vi "PH_Beckhoff_PP_Control.handle PP Mercury.vi"(0 "i ref in":refnum<vi>, 1 "changed DE Values":i32[](array[numeric]), 2 "changed AE Values":i32[](array[numeric]), 3 "Current Digital Inputs":T3, 4 "Current Analog Inputs":T1, 5 "error in":errorcluster) -> (14 "i ref out":refnum<vi>, 19 "error out":errorcluster)   [LabVIEW 2014, in "PH_Beckhoff_PP_Control.lvlib"]
doc: "This VI handles all information related to the PP mercury measurement. If it changed, it publishes the current status, the time since running, and sets the related GUI element."
uses:
  PH_Beckhoff_PP_Control.lvlib
  PH_Beckhoff/PH_Beckhoff.Digital Inputs.ctl
  PH_Beckhoff/PH_Beckhoff.Analog Inputs.ctl
  PH_Beckhoff/PH_Beckhoff.Scaling Type.ctl
  PH_StatusHandler/PH_StatusHandler.Status.ctl
  PH_StatusHandler/PH_StatusHandler.lvlib
  lib.lib/DimLVEvent/LVDimInterface/LVDimInterface.lvlib
  PH_Common/PH_Common.lvlib
  PH_Beckhoff/PH_Beckhoff.lvlib
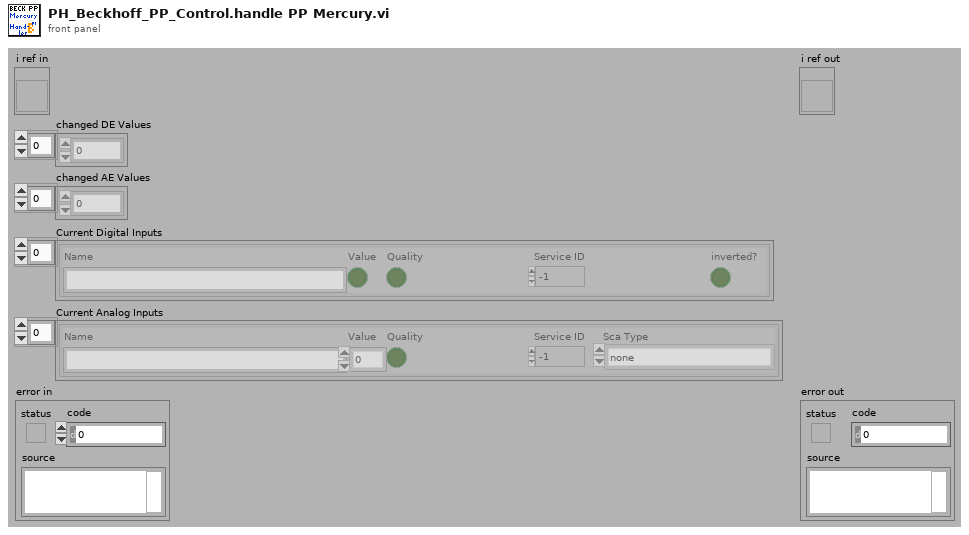
[diagram p1: front panel]
types:
  T1 = typedef "PH_Beckhoff.lvlib/PH_Beckhoff.Analog Inputs.ctl" = cluster{"Name":string, "Value":u32, "Quality":bool, "Service ID":i32, "Sca Type":T2}[]
  T2 = typedef "PH_Beckhoff.lvlib/PH_Beckhoff.Scaling Type.ctl" = enum16{"none", "0 ... 15 Bit -> 0 ... 5", "0 ... 15 Bit -> 0 ... 10", "0 ... 15 Bit -> 0 ... 25", "0 ... 15 Bit -> 4 ... 20", "0 ... 15 Bit -> 0 ... 1", "0 ... 15 Bit -> 0 ... 20000", "0 ... 15 Bit -> 0 ... 24000"}
  T3 = typedef "PH_Beckhoff.lvlib/PH_Beckhoff.Digital Inputs.ctl" = cluster{"Name":string, "Value":bool, "Quality":bool, "Service ID":i32, "inverted?":bool}[]
  T4 = typedef "PH_Beckhoff_PP_Control.lvlib/PH_Beckhoff_PP_Control.i attribute.ctl" = cluster{"PP Conductivity Control":cluster{"PSDB":cluster{"Status Service ID":i32, "Instance ID":i32, "Data Status":T5, "Ref Status":refnum<vi>, "Error Code":i32}, "Status":cluster{"GUI Ref":refnum<vi>, "Status Service ID":i32, "Status":T6}, "DIs":cluster{"Device on":cluster{"GUI Ref":refnum<vi>, "# in Data":i32}, "Conductivity ok":cluster{"GUI Ref":refnum<vi>, "# in Data":i32}, "Temperature ok":cluster{"GUI Ref":refnum<vi>, "# in Data":i32}, "Alarm":cluster{"GUI Ref":refnum<vi>, "# in Data":i32}}, "PSDB Thread":cluster{"Ref":refnum<vi>, "Q-Ref":refnum<queue>}}, "PP Mercury Control":cluster{"PSDB":cluster{"Status Service ID":i32, "Instance ID":i32, "Data Status":T5, "Ref Status":refnum<vi>, "Error Code":i32}, "Status":cluster{"GUI Ref":refnum<vi>, "Status Service ID":i32, "Status":T6}, "on since:":cluster{"GUI Ref":refnum<vi>, "Service ID":i32, "Time":string}, "DIs":cluster{"Device on":cluster{"GUI Ref":refnum<vi>, "# in Data":i32}, "Alarm":cluster{"GUI Ref":refnum<vi>, "# in Data":i32}}, "AIs":cluster{"Concentration":cluster{"GUI Ref":refnum<vi>, "# in Data":i32}}, "PSDB Thread":cluster{"Ref":refnum<vi>, "Q-Ref":refnum<queue>}}, "PSDB":cluster{"Shot #":i32, "Subsystem":T7}, "PSDB Credentials":T8}
  T5 = typedef "PH_PSDBWriter.lvlib/PH_PSDBWriter.Data Status.ctl" = i16
  T6 = typedef "PH_StatusHandler.lvlib/PH_StatusHandler.Status.ctl" = i16
  T7 = typedef "PH_PSDBWriter.lvlib/PH_PSDBWriter.PHELIX-Subsystems.ctl" = i32
  T8 = typedef "PH_Common.lvlib/PH_Connection.PSDB Credentials.ctl" = cluster{"PW":string, "ID":string, "DS":string}
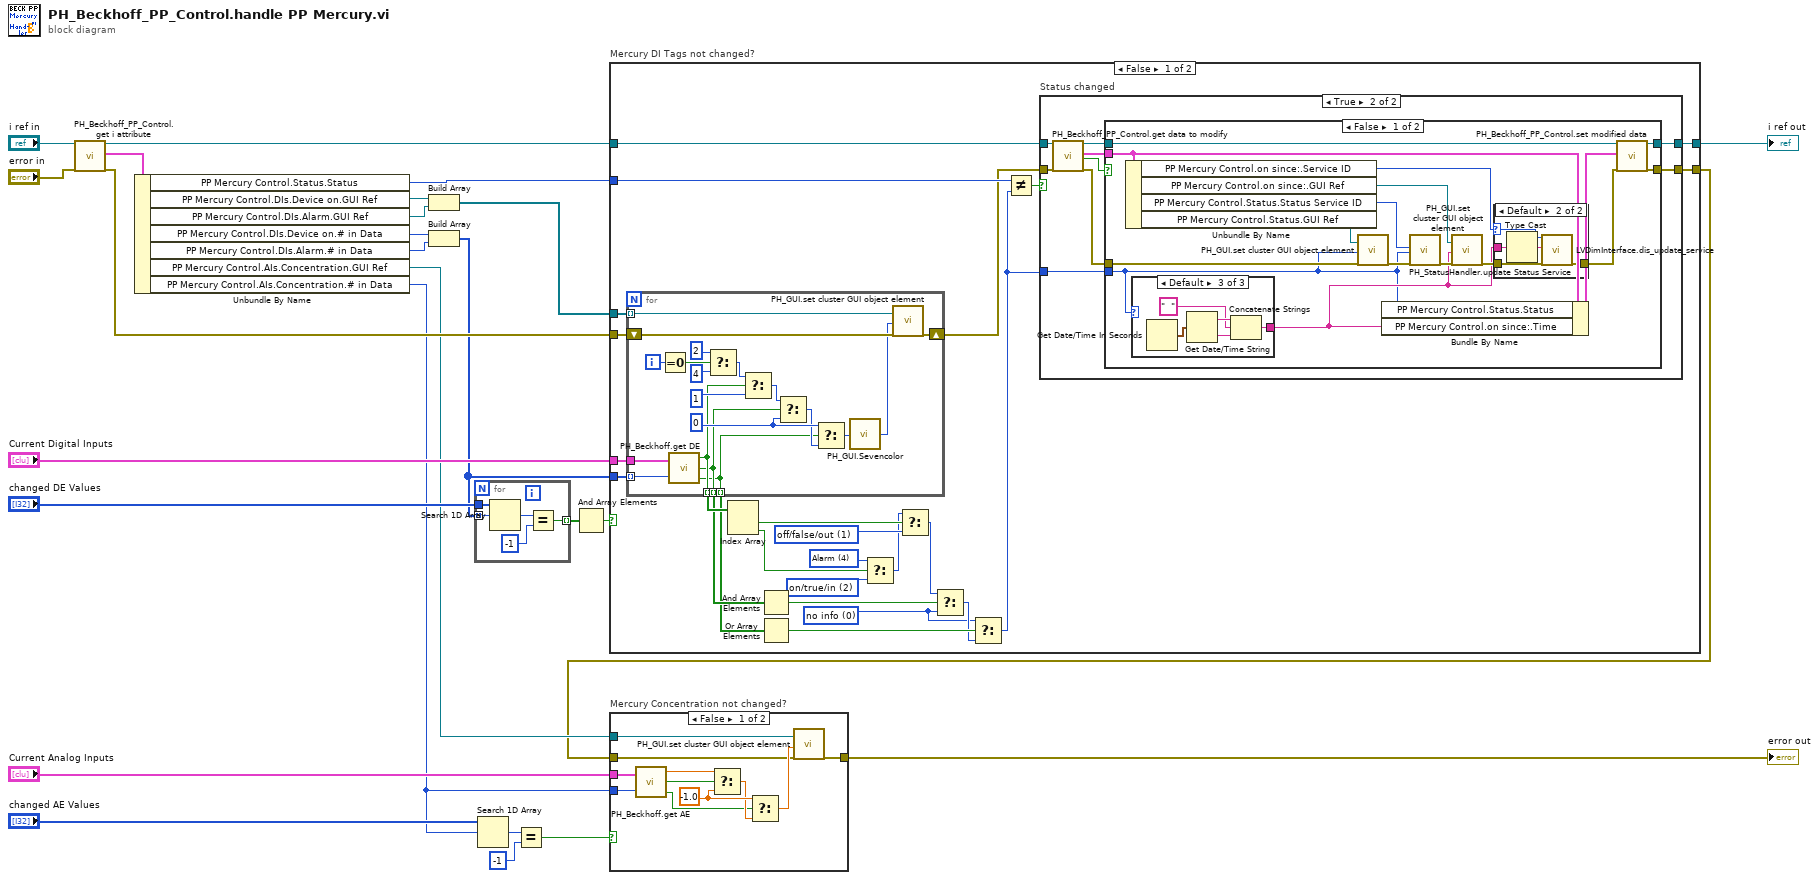
[diagram p0: block diagram]
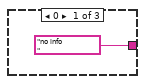
[diagram p5: hidden frame]
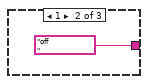
[diagram p6: hidden frame]
diagram:
  n1 = call "PH_Beckhoff_PP_Control.get i attribute.vi"("i ref in"="i ref in", "error in (no error)"="error in") -> ("i ref out"=w24:refnum<vi>, "i attribute"=w22:T4, "error out"=w13:errorcluster)  [unwired: 15 in]
  n2 = Unbundle By Name(w22) -> ("PP Mercury Control.Status.Status"=w21:T6, "PP Mercury Control.DIs.Device on.GUI Ref"=w18:refnum<vi>, "PP Mercury Control.DIs.Alarm.GUI Ref"=w17:refnum<vi>, "PP Mercury Control.DIs.Device on.# in Data"=w16:i32, "PP Mercury Control.DIs.Alarm.# in Data"=w15:i32, "PP Mercury Control.AIs.Concentration.GUI Ref"=w7:refnum<vi>, "PP Mercury Control.AIs.Concentration.# in Data"=w6:i32)
  n3 = Build Array(w18, w17) -> (w14:refnum<vi>[])
  n4 = Build Array(w16, w15) -> (w11:i32[])
  n5 = for {
    tunnel: "changed DE Values" -> [w31]
    tunnel: w11 -> [w30] mode=indexing
    tunnel: [w29] -> w10 mode=indexing
    n6 = Search 1D Array(1D array=w31, element=w30) -> (index of element=w28:i32)  [unwired: 1 in]
    n7 = Equal?(x=w28, y=-1) -> (x = y?=w29:bool)
  }
  n8 = Search 1D Array(1D array="changed AE Values", element=w6) -> (index of element=w2:i32)  [unwired: 1 in]
  n9 = Equal?(x=w2, y=-1) -> (x = y?=w3:bool)
  n10 = And Array Elements(Boolean array=w10) -> (logical AND=w9:bool)
  n11 = case "Mercury DI Tags not changed?" shown="False" w9 {
    tunnel: w24 -> [w43 w119]
    tunnel: w21 -> [w42 _]
    tunnel: [w41 w119] -> w20
    tunnel: [w40 w118] -> w5
    tunnel: "Current Digital Inputs" -> [w39 _]
    tunnel: w14 -> [w35 _]
    tunnel: w13 -> [w34 w118]
    tunnel: w11 -> [w32 _]
    frame False {
      w45 = T6 2 items=["no info", "off/false/out", "on/true/in", "Failure", "Alarm", "Status 1", "Status 2", "Status 3"] ("PP Mercury Control.Status")
      w46 = T6 4 items=["no info", "off/false/out", "on/true/in", "Failure", "Alarm", "Status 1", "Status 2", "Status 3"] ("PP Mercury Control.Status")
      w50 = T6 1 items=["no info", "off/false/out", "on/true/in", "Failure", "Alarm", "Status 1", "Status 2", "Status 3"] ("PP Mercury Control.Status")
      w52 = T6 0 items=["no info", "off/false/out", "on/true/in", "Failure", "Alarm", "Status 1", "Status 2", "Status 3"] ("PP Mercury Control.Status")
      n12 = for {
        shift-right: [w65] -> w33
        shift-left: w34 -> [w64]
        tunnel: w35 -> [w63] mode=indexing
        tunnel: w39 -> [w61]
        tunnel: [w60] -> w38 mode=indexing
        tunnel: [w59] -> w37 mode=indexing
        tunnel: [w58] -> w36 mode=indexing
        tunnel: w32 -> [w57] mode=indexing
        i -> [w70]
        w75 = 0 ("State")
        n13 = Equal To 0?(x=w70) -> (x = 0?=w69:bool)
        n14 = call "PH_Beckhoff.get DE.vi"("Digital Values"=w61, "index of element"=w57) -> ("Value"=w60:bool, "Quality"=w59:bool, "Tag not found"=w58:bool)
        n15 = Select(t=2 ("State"), s=w69, f=4) -> (s? t:f=w67:i32)
        n16 = Select(t=w67, s=w60, f=1 ("State")) -> (s? t:f=w71:i32)
        n17 = Select(t=w71, s=w59, f=w75) -> (s? t:f=w74:i32)
        n18 = Select(t=w75, s=w58, f=w74) -> (s? t:f=w73:i32)
        n19 = call "PH_GUI.Sevencolor.vi"("State"=w73) -> ("Color Box"=w62:u32)
        n20 = call "PH_GUI.set cluster GUI object element.vi"("Ctl Refnum"=w63, "Value"=w62, "error in"=w64) -> ("error out"=w65:errorcluster)  [unwired: 16 in]
      }
      n21 = Index Array(array=w38) -> (element #1=w51:bool, element #2=w48:bool)  [unwired: 2 in]
      n22 = And Array Elements(Boolean array=w37) -> (logical AND=w54:bool)
      n23 = Or Array Elements(Boolean array=w36) -> (logical OR=w55:bool)
      n24 = Select(t=w46, s=w48, f=w45) -> (s? t:f=w47:T6)
      n25 = Select(t=w47, s=w51, f=w50) -> (s? t:f=w49:T6)
      n26 = Select(t=w49, s=w54, f=w52) -> (s? t:f=w53:T6)
      n27 = Select(t=w52, s=w55, f=w53) -> (s? t:f=w44:T6)
      n28 = Not Equal?(x=w42, y=w44) -> (x != y?=w56:bool)
      n29 = case "Status changed" shown="True" w56 {
        tunnel: w33 -> [w76 w86]
        tunnel: [w76 w84] -> w40
        tunnel: w43 -> [w77 w83]
        tunnel: [w77 w81] -> w41
        tunnel: w44 -> [_ w78]
        frame False {
        }
        frame True {
          n30 = call "PH_Beckhoff_PP_Control.get data to modify.vi"("i ref in"=w83, "error in (no error)"=w86) -> ("i ref out"=w82:refnum<vi>, "i attribute"=w79:T4, "timed out"=w80:bool, "error out"=w85:errorcluster)  [unwired: 14 in]
          n31 = case shown="False" w80 {
            tunnel: w85 -> [w90 w116]
            tunnel: [w102 w116] -> w84
            tunnel: w82 -> [w101 w117]
            tunnel: [w100 w117] -> w81
            tunnel: w79 -> [w98 _]
            tunnel: w78 -> [w87 _]
            frame False {
              n32 = Unbundle By Name(w98) -> ("PP Mercury Control.on since:.Service ID"=w96:i32, "PP Mercury Control.on since:.GUI Ref"=w91:refnum<vi>, "PP Mercury Control.Status.Status Service ID"=w97:i32, "PP Mercury Control.Status.GUI Ref"=w88:refnum<vi>)
              n33 = case shown="Default" w87 {
                tunnel: ["no info                              " "off                                  " w112] -> w92
                frame 0 {
                }
                frame 1 {
                }
                frame Default {
                  n34 = Get Date/Time In Seconds() -> (seconds since 1Jan1904=w111:timestamp)
                  n35 = Get Date/Time String(seconds (now)=w111) -> (date string=w115:string, time string=w114:string)  [unwired: 2 in]
                  n36 = Concatenate Strings(w115, "  " ("string"), w114) -> (w112:string)
                }
              }
              n37 = call "PH_GUI.set cluster GUI object element.vi"("Ctl Refnum"=w88, "Value"=w87, "error in"=w90) -> ("error out"=w89:errorcluster)  [unwired: 16 in]
              n38 = Bundle By Name(cluster=w98, "PP Mercury Control.Status.Status"=w87, "PP Mercury Control.on since:.Time"=w92) -> (w99:T4)
              n39 = call "PH_StatusHandler.update Status Service.vi"("Service ID"=w97, "Status"=w87, "error in (no error)"=w89) -> ("error out"=w95:errorcluster)  [unwired: 16 in]
              n40 = call "PH_GUI.set cluster GUI object element.vi"("Ctl Refnum"=w91, "Value"=w92, "error in"=w95) -> ("error out"=w93:errorcluster)  [unwired: 16 in]
              n41 = case shown="Default" w96 {
                selector: w96 -> [_ w107]
                tunnel: [w103 w104] -> w94
                tunnel: w93 -> [w103 w108]
                tunnel: w92 -> [_ w105]
                frame -1 {
                }
                frame Default {
                  n42 = Type Cast(x=w105) -> (*(type *) &x=w106:string)  [unwired: 1 in]
                  n43 = call "LVDimInterface.dis_update_service.vi"("my_serviceID"=w107, "data"=w106, "error in (no error)"=w108) -> ("error out"=w104:errorcluster)  [unwired: 14 in, 2 out]
                }
              }
              n44 = call "PH_Beckhoff_PP_Control.set modified data.vi"("i ref in"=w101, "i attribute"=w99, "error in (no error)"=w94) -> ("i ref out"=w100:refnum<vi>, "error out"=w102:errorcluster)  [unwired: 15 in]
            }
            frame True {
            }
          }
        }
      }
    }
    frame True {
    }
  }
  "i ref out" <- w20
  n45 = case "Mercury Concentration not changed?" shown="False" w3 {
    tunnel: "Current Analog Inputs" -> [w130 _]
    tunnel: w7 -> [w123 _]
    tunnel: w6 -> [w122 _]
    tunnel: w5 -> [w121 w131]
    tunnel: [w120 w131] -> w4
    frame False {
      w129 = -1.0 ("t")
      n46 = call "PH_Beckhoff.get AE.vi"("Analog Inputs"=w130, "index of element"=w122) -> ("DIM value"=w127:dbl, "Quality"=w126:bool, "Tag not found"=w125:bool)
      n47 = Select(t=w127, s=w126, f=w129) -> (s? t:f=w128:dbl)
      n48 = Select(t=w129, s=w125, f=w128) -> (s? t:f=w124:dbl)
      n49 = call "PH_GUI.set cluster GUI object element.vi"("Ctl Refnum"=w123, "Value"=w124, "error in"=w121) -> ("error out"=w120:errorcluster)  [unwired: 16 in]
    }
    frame True {
    }
  }
  "error out" <- w4
